vi "about SQLDriverConnect.vi"(5 "error in (no error)":errorcluster, 7 "Database Path (empty)":path, 8 "InputHandle":i32) -> (0 "error out":errorcluster, 3 "OutputHandle":i32)   [LabVIEW 2011]
doc: "Se connecte auprès de la base spécifiée. S'identifie par le nom d'utilisateur et le mot de passe associé"
uses:
  Odbc32.dll
panel:
  out "OutConnectionString":string
  out "Overflow":i16
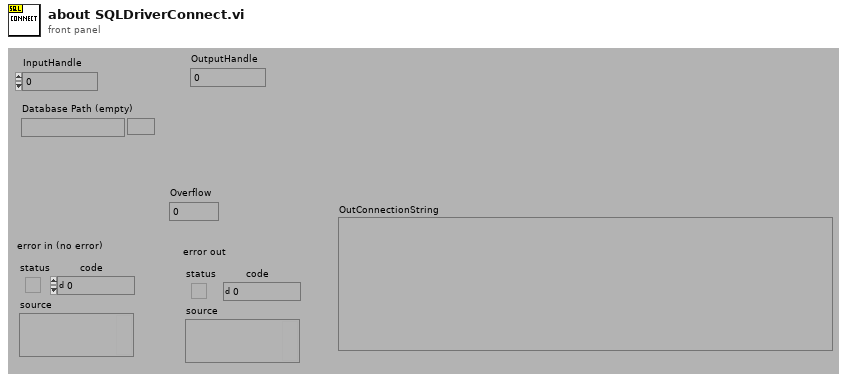
[diagram p1: front panel]
types:
  T1 = enum16{"NOPE", "SQL_HANDLE_ENV", "SQL_HANDLE_DBC", "SQL_HANDLE_STMT", "SQL_HANDLE_DESC"}
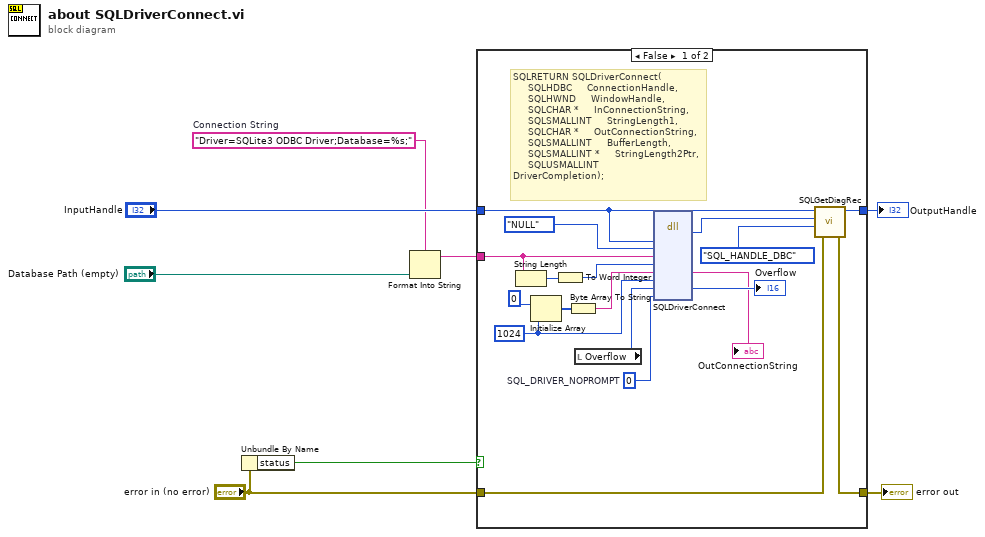
[diagram p0: block diagram]
diagram:
  w3 = "Driver=SQLite3 ODBC Driver;Database=%s;"  # Connection String
  n1 = Unbundle By Name("error in (no error)") -> ("status"=w7:bool)
  n2 = Format Into String(format string=w3, "Database Path (empty)") -> (resulting string=w1:string)  [unwired: 2 in, 1 out]
  n3 = case shown="False" w7 {
    tunnel: "InputHandle" -> [w26 w28]
    tunnel: "error in (no error)" -> [w24 w27]
    tunnel: [w23 w27] -> w6
    tunnel: [w25 w28] -> w5
    tunnel: w1 -> [w11 _]
    frame False {
      w14 = u16 0  # SQL_DRIVER_NOPROMPT
      w15 = i16 1024 ("dimension size")
      # "SQLRETURN SQLDriverConnect(\n     SQLHDBC     ConnectionHandle,\n     SQLHWND     WindowHandle,\n     SQLCHAR *     InConnectionString,\n     SQLSMALLINT     StringLength1,\n     SQLCHAR *     OutConnectionString,\n     SQLSMALLINT     BufferLength,\n     SQLSMALLINT *     StringLength2Ptr,\n     SQLUSMALLINT     DriverCompletion);"
      n4 = String Length(string=w11) -> (length=w19:i32)
      n5 = Initialize Array(u8 0, w15) -> (w16:u8[])
      n6 = To Word Integer(number=w19) -> (16bit integer=w18:i16)
      n7 = Byte Array To String(unsigned byte array=w16) -> (string=w9:string)
      n8 = local read "Overflow"() -> (w13:i16)
      n9 = dll-call lib="Odbc32.dll" fn="SQLDriverConnect"("ConnectionHandle"=w26, "WindowHandle"=enum32{"NULL"}."NULL", "InConnectionString"=w11, "StringLength1"=w18, "OutConnectionString"=w9, "BufferLength"=w15, "StringLength2Ptr"=w13, "DriverCompletion"=w14) -> ("SQLRETURN"=w22:i16, "OutConnectionString"=→"OutConnectionString":string, "StringLength2Ptr"=→"Overflow":i16)  [unwired: 8 in, 3 out]
      n10 = call "SQLGetDiagRec.vi"("error in (no error)"=w24, "HandleType"=T1."SQL_HANDLE_DBC", "Status (SQL_SUCCESS=0)"=w22, "Input Handle"=w26) -> ("error out"=w23:errorcluster, "Output Handle"=w25:i32)  [unwired: 2 out]
    }
    frame True {
    }
  }
  "OutputHandle" <- w5
  "error out" <- w6
